vi "Agilent SNA Filter Unmeasurable Measurements.vi"(7 "Agilent SNA & SWP":T5, 8 "error in (no error)":errorcluster, 10 "Parameters to Measure":T1[](array[typedef]) {"Channel" min=1 max=99 step=1; "Parameter"."Stimulus Port" min=1 step=1; "Parameter"."Response Port" min=1 step=1}, 11 "VISA Resource Names":T6) -> (0 "error out":errorcluster, 1 "Removed Parameters":T1[](array[typedef]) {"Channel" min=1 max=99 step=1; "Parameter"."Stimulus Port" min=1 step=1; "Parameter"."Response Port" min=1 step=1}, 2 "Filtered Parameters to Measure":T1[](array[typedef]) {"Channel" min=1 max=99 step=1; "Parameter"."Stimulus Port" min=1 step=1; "Parameter"."Response Port" min=1 step=1}, 3 "dup VISA Resource Names":T6, 4 "Measurements Removed?":bool)   [LabVIEW 2011]
uses:
  tests/S Parameter/TypeDefs/SP Parameter to Measure.ctl
  tests/S Parameter/TypeDefs/SP Parameter.ctl
  tests/S Parameter/TypeDefs/SP Calibration State.ctl
  tests/S Parameter/TypeDefs/SP Measurement Format.ctl
  TypeDefs/Agilent SNA VISA.ctl
  TypeDefs/Agilent SNA Instrument Info.ctl
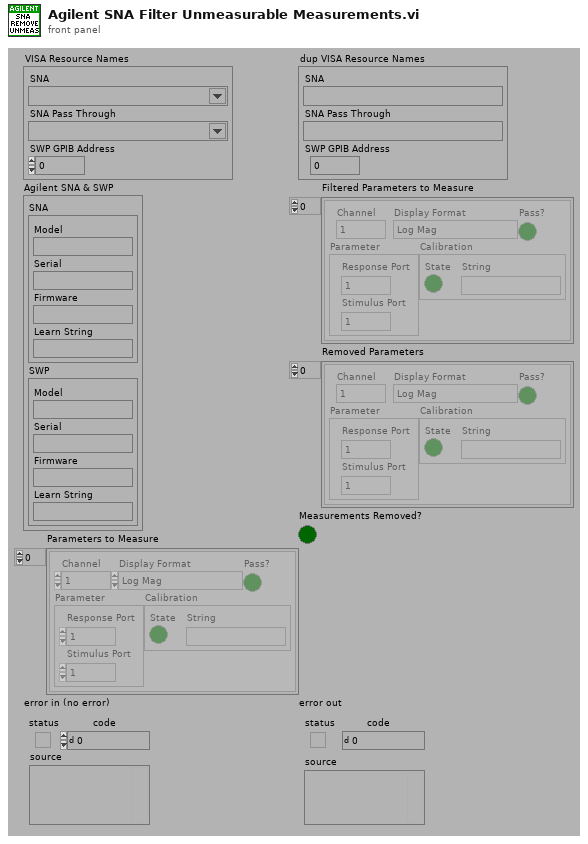
[diagram p1: front panel]
types:
  T1 = typedef "SP Parameter to Measure.ctl" = cluster{"Channel":i8, "Parameter":T2, "Calibration":T3, "Display Format":T4, "Pass?":bool}
  T2 = typedef "SP Parameter.ctl" = cluster{"Stimulus Port":i8, "Response Port":i8}
  T3 = typedef "SP Calibration State.ctl" = cluster{"State":bool, "String":string}
  T4 = typedef "SP Measurement Format.ctl" = enum32{"Log Mag", "Phase", "Delay", "Smith (R+jX)", "Polar (Re/Im)", "Linear Mag", "SWR", "Real", "Imaginary", "Smith (Lin/Phase)", "Smith (Log/Phase)", "Smith (Real/Imag)", "Smith (G+jB)", "Polar (Lin/Phase)", "Polar (Log/Phase)", "Expanded Phase", "Positive Phase", "Inverted Smith", "Unwrapped Phase", "Power Out", "Power In", "Linear Mag/Phase", "Log Mag/Phase", "Real/Imaginary"}
  T5 = typedef "Agilent SNA Instrument Info.ctl" = cluster{"SNA":cluster{"Model":string, "Serial":string, "Firmware":string, "Learn String":string}, "SWP":cluster{"Model":string, "Serial":string, "Firmware":string, "Learn String":string}}
  T6 = typedef "Agilent SNA VISA.ctl" = cluster{"SNA":refnum<visa-resource-name>, "SNA Pass Through":refnum<visa-resource-name>, "SWP GPIB Address":i32}
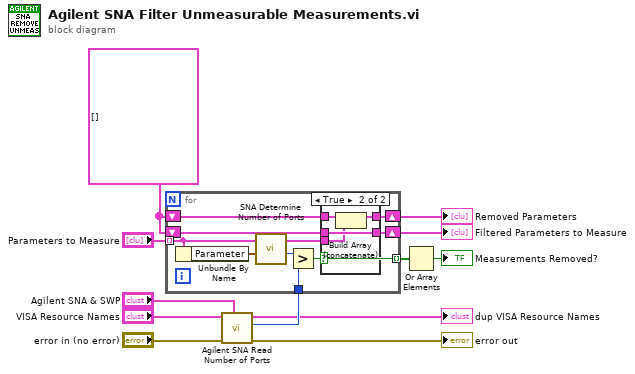
[diagram p0: block diagram]
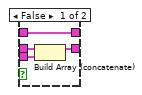
[diagram p2: hidden frame]
diagram:
  w2 = T1[] [] ("Parameters to Measure")
  n1 = call "Agilent SNA Read Number of Ports.vi"("Agilent SNA & SWP"="Agilent SNA & SWP", "error in (no error)"="error in (no error)", "VISA Resource Names"="VISA Resource Names") -> ("error out"=→"error out":errorcluster, "Number of Ports"=w8:i8, "dup VISA Resource Names"=→"dup VISA Resource Names":T6)  [unwired: 6 out]
  n2 = for {
    tunnel: "Parameters to Measure" -> [w17] mode=indexing
    shift-right: [w16] -> w5
    shift-left: w2 -> [w18]
    tunnel: w8 -> [w19]
    tunnel: [w15] -> w4 mode=indexing
    shift-right: [w13] -> w1
    shift-left: w2 -> [w14]
    n3 = Unbundle By Name(w17) -> ("Parameter"=w21:T2)
    n4 = call "SNA Determine Number of Ports.vi"("Parameter"=w21) -> ("Number of Ports"=w20:i8)  [unwired: 10 out]
    n5 = Greater?(x=w20, y=w19) -> (0:w15:bool)
    n6 = case shown="True" w15 {
      tunnel: w18 -> [w25 w29]
      tunnel: w17 -> [w24 w26]
      tunnel: [w23 w29] -> w16
      tunnel: w14 -> [w22 w28]
      tunnel: [w22 w27] -> w13
      frame False {
        n7 = Build Array (concatenate)(w25, w24) -> (w23:T1[])
      }
      frame True {
        n8 = Build Array (concatenate)(w28, w26) -> (w27:T1[])
      }
    }
  }
  "Filtered Parameters to Measure" <- w5
  "Removed Parameters" <- w1
  n9 = Or Array Elements(Boolean array=w4) -> (logical OR=→"Measurements Removed?":bool)
